vi "4_5 Construct a VI Pro4.vi"() -> ()   [LabVIEW 2025]
panel:
  in  "stop":bool
  out "Right Number":bool
  out "Your Choice":i8
  in  "Guesse the right \nNumber from 1 to 5":i8
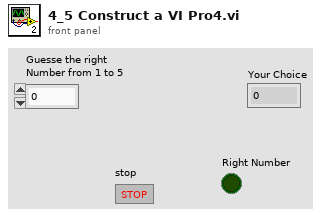
[diagram p1: front panel]
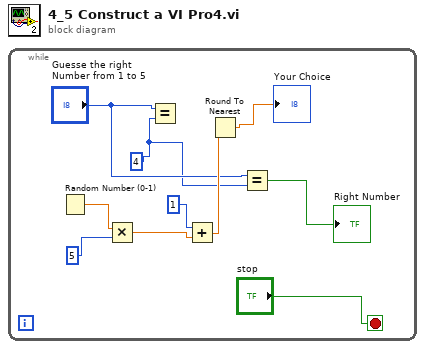
[diagram p0: block diagram]
diagram:
  n1 = while {
    stop <- "stop" stop-if-true
    w2 = 4
    n2 = Random Number (0-1)() -> (number: 0 to 1=w10:dbl)
    n3 = Multiply(x=w10, y=5) -> (x*y=w8:dbl)
    n4 = Equal?(x="Guesse the right \nNumber from 1 to 5", y=w2) -> ()  [unwired: 1 out]
    n5 = Add(x=1, y=w8) -> (x+y=w7:dbl)
    n6 = Round To Nearest(number=w7) -> (nearest integer value=→"Your Choice":dbl)
    n7 = Equal?(x="Guesse the right \nNumber from 1 to 5", y=w2) -> (x = y?=→"Right Number":bool)
  }
